vi "HFRR ADV v03.vi"() -> ()   [LabVIEW 2025] (continued)
              n1922 = local write "CH-POWER +"(w2879) -> ()
            }
            frame 12 {
              n1923 = local write "CH-POWER -"(w2880) -> ()
            }
            frame 13 {
              n1924 = local write "CH-HEATER"(w2881) -> ()
            }
            frame 14 {
              n1925 = local write "CH-HUMIDITY WET"(w2882) -> ()
            }
            frame 15 {
              n1926 = local write "CH-HUMIDITY DRY"(w2883) -> ()
            }
            frame 16 {
              n1927 = local read "Stroke PID Gains"() -> (w2886:T5)
              n1928 = Bundle By Name(cluster=w2886, "Integral Time (Ti, min)"=w2884) -> (w2885:T5)
              n1929 = local write "Stroke PID Gains"(w2885) -> ()
            }
            frame 17 {
              n1930 = local write "AIR TEMP INTERCEPT:"(w2887) -> ()
            }
            frame 18 {
              n1931 = local write "TEMP INTERCEPT:"(w2888) -> ()
            }
            frame 19 {
              n1932 = local write "S.NO"(w2889) -> ()
            }
            frame 20 {
              n1933 = local write "Com Port 3"(w2890) -> ()
            }
            frame 21 {
              n1934 = local write "LvdtOff"(w2891) -> ()
            }
            frame 22, Default {
            }
          }
        }
      }
    }
    n1935 = case shown="True" w2833 {
      frame False {
        # "79.77669138"
        # "2.3554"
        n1936 = local read "FRIC. FORCE :"() -> (w2896:dbl)
        n1937 = local read "FF cal val"() -> (w2893:dbl[])
        n1938 = Multiply(x=w2896, y=79.77669138) -> (x*y=w2895:dbl)
        n1939 = Multiply(x=w2893, y=w2895) -> (x*y=→"FF Calibration g":dbl[])
        "Err Count" <- 0 ("y")
      }
      frame True {
        n1940 = stacked-sequence {
          frame #0 {
            n1941 = stacked-sequence {
              frame #0 {
                "Lift" <- TRUE ("Lift")
              }
            }
          }
          frame #1 {
            w2908 = 2500 ("y")
            n1942 = local read "FF1"() -> (w2903:dbl[])
            n1943 = local read "Ch1"() -> (w2899:dbl[])
            "Waveform Chart 2" <- w2899
            n1944 = Array Size(array=w2903) -> (size(s)=w2902:i32)
            n1945 = Insert Into Array(array=w2903, index=w2902, new element=w2899) -> (w2905:dbl[])
            n1946 = call-poly <vilib>:"Mean.vi"("X"=w2899) -> ("mean"=→"Raw Mean":dbl)  [unwired: 1 out]
            n1947 = local read "RUN"() -> (w2900:bool)
            n1948 = Array Size(array=w2905) -> (size(s)=w2909:i32)
            n1949 = case shown="False" w2900 {
              frame False {
                n1950 = local write "Frequency"(0.0 ("Frequency")) -> ()
              }
              frame True {
              }
            }
            n1951 = Subtract(x=w2909, y=w2908) -> (x-y=w2907:i32)
            n1952 = Greater?(x=w2909, y=w2908) -> (0:w2910:bool)
            n1953 = case shown="True" w2910 {
              tunnel: w2907 -> [_ w2914]
              tunnel: [w2912 w2916] -> w2901
              tunnel: w2905 -> [w2912 w2915]
              frame False {
              }
              frame True {
                n1954 = Delete From Array(array=w2915, length=w2914, index=0) -> (array with subset deleted=w2916:dbl[])  [unwired: 1 out]
                "Numeric" <- w2914
              }
            }
            "FF1" <- w2901
            "PID Ref" <- TRUE ("PID Ref")
          }
          frame #2 {
          }
          frame #3 {
            w2917 = 0.0 ("lower limit")
            w2949 = 0.0 ("lower limit")
            # "CONVERT TO N"
            # "DATA PROCESSING"
            # "115 mV/N"
            n1955 = local read "Fric Val"() -> (w3010:dbl[])
            n1956 = local read "FRIC. FORCE :"() -> (w3000:dbl)
            n1957 = local read "Air temp"() -> (w3001:dbl[])
            n1958 = local read "temp buf"() -> (w3004:dbl[])
            n1959 = call-poly <vilib>:"Mean.vi"("X"=w3001) -> ("mean"=w2941:dbl)  [unwired: 1 out]
            "Raw air temp" <- w2941
            n1960 = local read "humid"() -> (w2951:string)
            n1961 = Multiply(x=w3010, y=1.0) -> (x*y=w3011:dbl[])
            n1962 = Multiply(x=w3000, y=79.77669138) -> (x*y=w2998:dbl)
            n1963 = call-poly <vilib>:"Mean.vi"("X"=w3004) -> ("mean"=w2943:dbl)  [unwired: 1 out]
            "Raw specimen temp" <- w2943
            n1964 = case shown="0, Default" "Calibrating" {
              tunnel: w2943 -> [w3033 _]
              tunnel: [w3033 w3034] -> w2942
              tunnel: w2941 -> [_ w3034]
              frame 0, Default {
              }
              frame 1 {
              }
            }
            n1965 = local read "HUMIDITY:"() -> (w3014:dbl)
            n1966 = Multiply(x=w3011, y=w2998) -> (x*y=w3008:dbl[])
            n1967 = Add(x=w2941, y="Offset Air Temp") -> (x+y=w2936:dbl)
            n1968 = local read "AIR TEMPERATURE :"() -> (w2985:dbl)
            n1969 = Fract/Exp String To Number(string=w2951) -> (number=w2950:dbl)  [unwired: 3 in, 1 out]
            n1970 = local read "TEMPERATURE :"() -> (w2984:dbl)
            n1971 = call-poly <vilib>:"Mean.vi"("X"=w3008) -> ("mean"=w3009:dbl)  [unwired: 1 out]
            n1972 = Multiply(x=w2950, y=w3014) -> (x*y=w3006:dbl)
            n1973 = Subtract(x=w3008, y=w3009) -> (x-y=w2947:dbl[])
            n1974 = case shown="True" "Boolean 4" {
              tunnel: w2942 -> [_ w3040]
              tunnel: "Standard Temp. ( °c )" -> [_ w3039]
              frame False {
              }
              frame True {
                n1975 = local read "Captured Values"() -> (w3037:dbl[][])
                n1976 = local write "Boolean 4"(FALSE ("Boolean 4")) -> ()
                n1977 = Build Array(w3039, w3040) -> (w3038:dbl[])
                n1978 = Build Array (concatenate)(w3037, w3038) -> (w3035:dbl[][])
                n1979 = local write "Captured Values"(w3035) -> ()
              }
            }
            n1980 = local read "AIR TEMP INTERCEPT:"() -> (w2981:dbl)
            n1981 = Multiply(x=w2936, y=w2985) -> (x*y=w2938:dbl)
            n1982 = Absolute Value(x=w2947) -> (abs(x)=w3015:dbl[])
            n1983 = Multiply(x=w2943, y=w2984) -> (x*y=w2937:dbl)
            n1984 = In Range and Coerce(upper limit=100.0, x=w3006, lower limit=w2949) -> (coerced(x)=w2953:dbl)  [unwired: 1 out]
            n1985 = local read "TEMP INTERCEPT:"() -> (w2948:dbl)
            n1986 = local read "Humid Last buf"() -> (w2976:dbl[])
            n1987 = call-poly <vilib>:"RMS.vi"("X"=w2947) -> ("rms value"=w2946:dbl)  [unwired: 1 out]
            n1988 = call-poly <vilib>:"Mean.vi"("X"=w3015) -> ()  [unwired: 2 out]
            n1989 = local read "RUN"() -> (w2997:bool)
            n1990 = Add(x=w2938, y=w2981) -> (x+y=w2983:dbl)
            n1991 = Add(x=w2937, y=w2948) -> (x+y=w2982:dbl)
            n1992 = local read "FRICVALZ"() -> (w3021:dbl)
            n1993 = Replace Array Subset(array=w2976, new element=w2953, index=0) -> (w2972:dbl[])
            n1994 = call <vilib>:"Mean PtByPt.vi"("x"=w2982, "sample length"=10) -> ("mean"=w3002:dbl)  [unwired: 2 in, 1 out]
            "TEMP 2" <- w3002
            n1995 = Select(t=0.01 ("FF fil1"), s=w2997, f=0.1 ("FF fil1")) -> (s? t:f=w2993:dbl)
            n1996 = case shown="True" "FRICVALZ 2" {
              tunnel: w2946 -> [_ w3057]
              frame False {
              }
              frame True {
                n1997 = local write "FRICVALZ 2"(FALSE ("FRICVALZ")) -> ()
                "FRICVALZ" <- w3057
              }
            }
            n1998 = Subtract(x=w2946, y=w3021) -> (x-y=w3012:dbl)
            n1999 = local read "AIR TEMP"() -> (w2990:dbl)
            n2000 = Multiply(x=w2983, y=w2993) -> (x*y=w2994:dbl)
            n2001 = Subtract(x=w2953, y=w2949) -> (x-y=w2952:dbl)
            "Humidity ( Rh )" <- w2952
            n2002 = Rotate 1D Array(1:w2972, 2:1 ("n")) -> (0:w2973:dbl[])
            n2003 = Index Array(array=w2972, index #1=0 ("index"), index #2=3 ("index")) -> (element #1=w2961:dbl, element #2=w2960:dbl)
            n2004 = case shown="True" "Boolean 5" {
              frame False {
              }
              frame True {
                n2005 = local write "Captured Values"(dbl[][] [] ("Captured Values")) -> ()
                n2006 = local write "Boolean 5"(FALSE) -> ()
                n2007 = local write "Best Fit"(dbl[] [] ("Best Fit")) -> ()
              }
            }
            n2008 = local read "FF 2"() -> (w3023:dbl)
            n2009 = Subtract(x=1.0 ("y"), y=w2993) -> (x-y=w2991:dbl)
            n2010 = Divide(x=w2961, y=w2960) -> (x/y=w2968:dbl)
            n2011 = Multiply(x=w2991, y=w2990) -> (x*y=w2989:dbl)
            n2012 = Multiply(x=w3012, y=0.1 ("FF fil1")) -> (x*y=w3027:dbl)
            n2013 = local write "TEMP"(w3002) -> ()
            n2014 = Multiply(x=0.9 ("FF fil2"), y=w3023) -> (x*y=w3026:dbl)
            n2015 = local write "Humid Last buf"(w2973) -> ()
            n2016 = Add(x=w2994, y=w2989) -> (x+y=w2987:dbl)
            n2017 = local read "offfset corr"() -> (w2964:bool)
            n2018 = local read "ecr buf"() -> (w2934:dbl[])
            n2019 = Subtract(x=1.0, y=w2968) -> (x-y=w2967:dbl)
            n2020 = Add(x=w3027, y=w3026) -> (x+y=w3020:dbl)
            "FF 2" <- w3020
            n2021 = local read "NORMAL LOAD"() -> (w3007:dbl)
            n2022 = Not A Number/Path/Refnum?(number/path/refnum=w2987) -> (NaN/Path/Refnum?=w2988:bool)
            n2023 = Absolute Value(x=w2967) -> (abs(x)=w2966:dbl)
            n2024 = Not(x=w2964) -> (.not. x?=w2962:bool)
            n2025 = Select(t=0.0, s=w2988, f=w2987) -> (s? t:f=w2919:dbl)
            "AIR TEMP" <- w2919
            n2026 = Greater Or Equal?(x=w2966, y=0.05) -> (x >= y?=w2955:bool)
            n2027 = call-poly <vilib>:"Mean.vi"("X"=w2934) -> ("mean"=w2931:dbl)  [unwired: 1 out]
            n2028 = And(x=w2955, y=w2962) -> (x .and. y?=w2963:bool)
            n2029 = Not A Number/Path/Refnum?(number/path/refnum=w2952) -> (NaN/Path/Refnum?=w3013:bool)
            n2030 = case shown="True" w3013 {
              frame False {
              }
              frame True {
                n2031 = local write "Humidity ( Rh )"(0.0 ("Humidity 3")) -> ()
              }
            }
            n2032 = case shown="True" w2963 {
              tunnel: w2961 -> [_ w3051]
              tunnel: w2960 -> [_ w3050]
              frame False {
                w3045 = 5.0 ("y")
                n2033 = local read "cnter"() -> (w3047:dbl)
                n2034 = Increment(x=w3047) -> (x+1=w3044:dbl)
                n2035 = Greater Or Equal?(x=w3044, y=w3045) -> (x >= y?=w3046:bool)
                n2036 = Select(t=w3045, s=w3046, f=w3044) -> (s? t:f=w3043:dbl)
                n2037 = local write "cnter"(w3043) -> ()
              }
              frame True {
                n2038 = Subtract(x=w3051, y=w3050) -> (x-y=→"offset":dbl)
                "offfset corr" <- TRUE ("offfset corr")
                "cnter" <- 0.0 ("cnter")
              }
            }
            n2039 = Multiply(x=w2931, y="ECR_Gain") -> (x*y=w2930:dbl)
            n2040 = local read "TEMP"() -> (w3019:dbl)
            n2041 = local read "ecr"() -> (w2925:dbl)
            n2042 = Divide(x=w3020, y=w3007) -> (x/y=w2977:dbl)
            n2043 = local read "offfset corr"() -> (w2957:bool)
            n2044 = Multiply(x=w2930, y=0.2) -> (x*y=w2923:dbl)
            n2045 = Multiply(x=0.8, y=w2925) -> (x*y=w2924:dbl)
            n2046 = call "Elapsed Time11"("Time Target (s)"=1.0) -> ("Time has Elapsed"=w2921:bool)  [unwired: 11 in, 7 out]
            n2047 = local read "cnter"() -> (w2959:dbl)
            n2048 = Not A Number/Path/Refnum?(number/path/refnum=w3019) -> (NaN/Path/Refnum?=w3018:bool)
            n2049 = Not A Number/Path/Refnum?(number/path/refnum=w3020) -> (NaN/Path/Refnum?=w3017:bool)
            n2050 = Not A Number/Path/Refnum?(number/path/refnum=w2977) -> (NaN/Path/Refnum?=w2979:bool)
            n2051 = Add(x=w2923, y=w2924) -> (x+y=w2922:dbl)
            n2052 = Select(t=0.0, s=w2979, f=w2977) -> (s? t:f=→"COF 2":dbl)
            n2053 = case shown="True" w2921 {
              tunnel: w2919 -> [_ w3029]
              frame False {
              }
              frame True {
                "AirT" <- w3029
              }
            }
            n2054 = Equal?(x=5.0 ("y"), y=w2959) -> (x = y?=w2958:bool)
            n2055 = Compound Arithmetic op=OR(w3018, w3017) -> (w3016:bool)
            n2056 = Not A Number/Path/Refnum?(number/path/refnum=w2922) -> (NaN/Path/Refnum?=w2932:bool)
            n2057 = Compound Arithmetic op=AND(w2955, w2958, w2957) -> (w2954:bool)
            n2058 = case shown="True" w3016 {
              frame False {
              }
              frame True {
                n2059 = local write "TEMP"(0.0 ("TEMP")) -> ()
                n2060 = local write "reinit"(TRUE ("reinit")) -> ()
                n2061 = local write "FF 2"(0.0 ("FF 2")) -> ()
              }
            }
            n2062 = Select(t=0.0, s=w2932, f=w2922) -> (s? t:f=w2929:dbl)
            n2063 = case shown="True" w2954 {
              frame False {
              }
              frame True {
                n2064 = local write "offfset corr"(FALSE ("offfset corr")) -> ()
                n2065 = local write "offset"(0.0 ("offset")) -> ()
              }
            }
            n2066 = In Range and Coerce(upper limit=100.0, x=w2929, lower limit=w2917) -> ()  [unwired: 2 out]
            "ecr" <- w2917
          }
          frame #4 {
            n2067 = case shown="True" "Boolean 6" {
              frame False {
              }
              frame True {
                n2068 = local read "Captured Values"() -> (w3069:dbl[][])
                n2069 = Index Array(array=w3069, index (col) #1=0 ("disabled index (col)"), index (col) #2=1 ("index (col)")) -> (element #1=w3067:dbl[], element #2=w3065:dbl[])  [unwired: 2 in]
                n2070 = local write "Boolean 6"(FALSE ("Boolean 6")) -> ()
                n2071 = call <vilib>:"Linear Fit.vi"("Y"=w3067, "X"=w3065) -> ("Best Linear Fit"=→"Best Fit":dbl[], "slope"=w3061:dbl, "intercept"=w3060:dbl)  [unwired: 9 in, 2 out]
                "Slope" <- w3061
                "Intercept" <- w3060
                n2072 = local read "Calibrating"() -> (w3062:u16)
                n2073 = case shown="1" w3062 {
                  tunnel: w3061 -> [w3071 w3073]
                  tunnel: w3060 -> [w3070 w3072]
                  frame 0, Default {
                    n2074 = local write "TEMPERATURE :"(w3071) -> ()
                    n2075 = local write "TEMP INTERCEPT:"(w3070) -> ()
                  }
                  frame 1 {
                    n2076 = local write "AIR TEMPERATURE :"(w3073) -> ()
                    n2077 = local write "AIR TEMP INTERCEPT:"(w3072) -> ()
                  }
                }
              }
            }
            n2078 = flat-sequence {
              frame #0 {
                n2079 = Wait (ms)(milliseconds to wait=u32 100) -> ()  [unwired: 1 out]
              }
              frame #1 {
                n2080 = local write "Lift"(FALSE ("Lift")) -> ()
              }
            }
          }
        }
      }
    }
    n2081 = local read "EXIT"() -> (w2840:bool)
    "Rate" <- 2500.0 ("No of Samples")
    "Humid Last buf" <- dbl[] [0.0, 0.0, 0.0, 0.0] ("Humid Last buf")
  }
  n2082 = VISA Close(VISA resource name=w19, error in (no error)=w18) -> (error out=w20:errorcluster)
  n2083 = call <vilib>:"Clear Errors.vi"("error in (no error)"=w20) -> ()  [unwired: 5 in, 2 out]
  n2084 = VISA Close(VISA resource name=w47, error in (no error)=w46) -> (error out=w44:errorcluster)
  n2085 = call <vilib>:"Clear Errors.vi"("error in (no error)"=w44) -> ()  [unwired: 5 in, 2 out]
  n2086 = Or(x=w34, y=w33) -> (x .or. y?=w35:bool)
  n2087 = while {
    tunnel: [w3135] -> w40
    shift-right: [w3115] -> _
    shift-left: "" -> [w3103]
    tunnel: [w3091] -> _
    i -> [w3091]
    stop <- w3135 stop-if-true
    w3117 = ";" ("string")
    n2088 = local read "start en"() -> (w3137:bool)
    n2089 = And(x="st enable", y=w3137) -> (x .and. y?=w3138:bool)
    n2090 = local read "ACQUIRE 3"() -> (w3080:bool)
    n2091 = local read "Elapsed time"() -> (w3099:dbl)
    n2092 = case shown="True" w3138 {
      tunnel: "st enable" -> [w3202 w3203]
      tunnel: [w3202 w3203] -> w3081
      frame False {
      }
      frame True {
        n2093 = local write "start en"(FALSE ("start en")) -> ()
      }
    }
    n2094 = Wait (ms)(milliseconds to wait=u32 80) -> ()  [unwired: 1 out]
    n2095 = local read "Stroke"() -> (w3090:dbl)
    n2096 = Greater?(x=w3099, y=0.1) -> (0:w3097:bool)
    n2097 = Or(x=w3081, y=w3080) -> (x .or. y?=w3082:bool)
    n2098 = case shown="True" "ACQUIRE 2" {
      frame False {
      }
      frame True {
        n2099 = call "Elapsed Time13"() -> ("Time has Elapsed"=w3145:bool)  [unwired: 12 in, 7 out]
        n2100 = case shown="True" w3145 {
          frame False {
          }
          frame True {
            n2101 = local write "ACQUIRE 2"(FALSE ("ACQUIRE 2")) -> ()
            n2102 = local write "ACQUIRE 3"(FALSE ("ACQUIRE 2")) -> ()
          }
        }
        n2103 = local write "ACQUIRE 3"(TRUE ("ACQUIRE 2")) -> ()
      }
    }
    n2104 = case shown="True" w3082 {
      tunnel: w3090 -> [_ w3225]
      tunnel: [w3205 _] -> w3134
      tunnel: w3097 -> [_ _]
      tunnel: w3080 -> [_ w3212]
      frame False {
        w3205 = TRUE ("PID Rst")
        n2105 = local read "stop cmd"() -> (w3206:bool)
        n2106 = case shown="True" w3206 {
          frame False {
          }
          frame True {
            n2107 = local write "stop cmd"(FALSE ("stop cmd")) -> ()
          }
        }
        n2108 = local write "PID Rst"(TRUE ("PID Rst")) -> ()
        "start en" <- w3205
      }
      frame True {
        w3232 = cluster{"output high":dbl, "output low":dbl} {"output high"=600.0, "output low"=-600.0} ("output range")
        n2109 = local read "STROKE GAIN :"() -> (w3217:dbl)
        n2110 = call "Elapsed Time6"("Reset"="PID Rst", "Auto Reset"=FALSE) -> ("Time has Elapsed"=w3226:bool)  [unwired: 10 in, 7 out]
        n2111 = Multiply(x="Set Strk", y=w3217) -> (x*y=w3210:dbl)
        n2112 = case shown="False" w3226 {
          tunnel: [w3237 w3238] -> w3229
          tunnel: "Set Strk" -> [w3237 _]
          tunnel: w3225 -> [_ w3238]
          frame False {
          }
          frame True {
          }
        }
        n2113 = Multiply(x=w3210, y=1.0) -> (x*y=w3209:dbl)
        n2114 = Select(t=T5 {"Proportional Gain (Kc)"=0.0, "Integral Time (Ti, min)"=0.02, "Derivative Time (Td, min)"=0.0} ("Stroke PID Gains"), s=w3212, f="Stroke PID Gains") -> (s? t:f=w3213:T5)
        n2115 = Not(x=w3226) -> (.not. x?=w3224:bool)
        n2116 = call-poly <vilib>:"PID.vi"("reinitialize? (F)"=w3224, "output range"=w3232, "PID gains"=w3213, "process variable"=w3229, "setpoint"="Set Strk") -> ("output"=w3223:dbl)  [unwired: 5 in, 1 out]
        "Slide 5" <- w3223
        n2117 = Select(t=w3223, s=w3226, f=0.0) -> (s? t:f=w3227:dbl)
        n2118 = flat-sequence {
          tunnel: w3227 -> [_]
          frame #0 {
            n2119 = local write "PID Rst"(FALSE ("PID Rst")) -> ()
          }
        }
        n2120 = Add(x=w3209, y=w3227) -> (x+y=w3222:dbl)
        n2121 = Unbundle(w3232) -> ("output high"=w3231:dbl, "output low"=w3230:dbl)
        n2122 = To Word Integer(number=w3222) -> (16bit integer=w3219:i16)
        n2123 = property on="Slide 5" class="Slide (strict)"("Scale.Range:Minimum"=w3230, "Scale.Range:Maximum"=w3231) -> ()  [unwired: 2 in, 2 out]
        n2124 = In Range and Coerce(upper limit=4095.0 ("f"), x=w3219, lower limit=100.0 ("f")) -> (coerced(x)=w3216:dbl)  [unwired: 1 out]
        "PID Out" <- w3216
        n2125 = Number To Decimal String(number=w3216) -> (decimal integer string=→"st gain":string)  [unwired: 1 in]
        "stop cmd" <- TRUE ("Auto Reset")
      }
    }
    n2126 = flat-sequence {
      frame #0 {
        n2127 = local read "CH-POWER +"() -> (w3149:u16)
        n2128 = local read "CH-POWER -"() -> (w3150:u16)
        n2129 = case shown="1" w3150 {
          tunnel: "PWR" -> [w3151 w3152 w3153 w3154 w3155 w3156 w3157 w3158]
          frame 0, Default {
            n2130 = local write "Do 0"(w3151) -> ()
          }
          frame 1 {
            n2131 = local write "Do 1"(w3152) -> ()
          }
          frame 2 {
            n2132 = local write "Do 2"(w3153) -> ()
          }
          frame 3 {
            n2133 = local write "Do 3"(w3154) -> ()
          }
          frame 4 {
            n2134 = local write "Do 4"(w3155) -> ()
          }
          frame 5 {
            n2135 = local write "Do 5"(w3156) -> ()
          }
          frame 6 {
            n2136 = local write "Do 6"(w3157) -> ()
          }
          frame 7 {
            n2137 = local write "Do 7"(w3158) -> ()
          }
        }
        n2138 = case shown="1" w3149 {
          tunnel: "PWR" -> [w3159 w3160 w3161 w3162 w3163 w3164 w3165 w3166]
          frame 0, Default {
            n2139 = local write "Do 0"(w3159) -> ()
          }
          frame 1 {
            n2140 = local write "Do 1"(w3160) -> ()
          }
          frame 2 {
            n2141 = local write "Do 2"(w3161) -> ()
          }
          frame 3 {
            n2142 = local write "Do 3"(w3162) -> ()
          }
          frame 4 {
            n2143 = local write "Do 4"(w3163) -> ()
          }
          frame 5 {
            n2144 = local write "Do 5"(w3164) -> ()
          }
          frame 6 {
            n2145 = local write "Do 6"(w3165) -> ()
          }
          frame 7 {
            n2146 = local write "Do 7"(w3166) -> ()
          }
        }
      }
    }
    n2147 = local read "RUN"() -> (w3088:bool)
    n2148 = Or(x=w3088, y="ACQUIRE 3") -> (x .or. y?=w3087:bool)
    n2149 = local read "Set Hz"() -> (w3105:dbl)
    n2150 = Select(t=w3105, s=w3087, f=0.0) -> (s? t:f=w3104:dbl)
    n2151 = local read "st gain"() -> (w3108:string)
    n2152 = local read "DO"() -> (w3109:string)
    n2153 = case shown="True" "Boolean 10" {
      frame False {
      }
      frame True {
        n2154 = local write "Tab Control 8"(enum32{"setup", "calibrate"}."calibrate" ("Tab Control 8")) -> ()
        n2155 = local write "Boolean 10"(FALSE ("Boolean 10")) -> ()
      }
    }
    n2156 = Number To Decimal String(number=w3104) -> (decimal integer string=w3107:string)  [unwired: 1 in]
    n2157 = case shown="True" "Boolean 11" {
      frame False {
      }
      frame True {
        n2158 = local write "Tab Control 8"(enum32{"setup", "calibrate"}."setup" ("Tab Control 8")) -> ()
        n2159 = local write "Boolean 11"(FALSE ("Boolean 11")) -> ()
      }
    }
    n2160 = String Length(string=w3108) -> (length=w3123:i32)
    n2161 = String Length(string=w3109) -> (length=w3111:i32)
    n2162 = String Length(string=w3107) -> (length=w3124:i32)
    n2163 = Subtract(x=4.0, y=w3123) -> (x-y=w3120:dbl)
    n2164 = Subtract(x=3.0, y=w3111) -> (x-y=w3114:dbl)
    n2165 = flat-sequence {
      tunnel: w3134 -> [_]
      frame #0 {
        n2166 = Build Array("Do 0", "Do 1", "Do 2", "Do 3", "Do 4", "Do 5", "Do 6", "Do 7") -> (w3193:bool[])
        n2167 = Boolean Array To Number(Boolean array=w3193) -> (number=w3191:u32)
        n2168 = Add(x=w3191, y=u32 0) -> (x+y=w3189:u32)
        n2169 = Number To Decimal String(number=w3189) -> (decimal integer string=→"DO":string)  [unwired: 1 in]
      }
    }
    n2170 = Subtract(x=3.0, y=w3124) -> (x-y=w3125:dbl)
    n2171 = Replace Substring(3:w3120, 4:w3108, 5:"0000" ("string")) -> (1:w3118:string)  [unwired: 1 in, 1 out]
    n2172 = Replace Substring(3:w3114, 4:w3109, 5:"000" ("string")) -> (1:w3110:string)  [unwired: 1 in, 1 out]
    n2173 = Replace Substring(3:w3125, 4:w3107, 5:"000" ("string")) -> (1:w3119:string)  [unwired: 1 in, 1 out]
    n2174 = Concatenate Strings("*" ("string"), w3119, w3117, w3118, w3117, w3110, "$" ("string")) -> (w3115:string)
    "Stroke_send_Val" <- w3115
    n2175 = local read "RUN"() -> (w3085:bool)
    n2176 = local read "ACQUIRE 3"() -> (w3084:bool)
    n2177 = local read "send"() -> (w3101:bool)
    n2178 = Not Equal?(x=w3103, y=w3115) -> (x != y?=w3116:bool)
    n2179 = Or(x=w3085, y=w3084) -> (x .or. y?=w3083:bool)
    n2180 = And(x=w3101, y=w3083) -> (x .and. y?=w3100:bool)
    n2181 = Or(x=w3116, y=w3100) -> (x .or. y?=w3094:bool)
    n2182 = case shown="False" w3083 {
      frame False {
        "send" <- TRUE ("send")
      }
      frame True {
      }
    }
    n2183 = call "Elapsed Time4"("Time Target (s)"=0.5) -> ("Time has Elapsed"=w3092:bool)  [unwired: 11 in, 7 out]
    n2184 = local read "Din"() -> (w3133:u8[])
    n2185 = Or(x=w3092, y=w3094) -> (x .or. y?=w3093:bool)
    n2186 = Index Array(array=w3133, index=0) -> (element=w3131:u8)
    n2187 = case shown="True" w3093 {
      tunnel: w3115 -> [_ w3170]
      frame False {
      }
      frame True {
        n2188 = local read "Due Com"() -> (w3171:string[])
        n2189 = Build Array (concatenate)(w3171, w3170) -> (→"Due Com":string[])
        n2190 = local write "send"(FALSE ("send")) -> ()
      }
    }
    n2191 = Number To Boolean Array(number=w3131) -> (Boolean array=w3130:bool[])
    n2192 = Array Size(array=w3130) -> (size(s)=w3129:i32)
    n2193 = Greater Than 0?(x=w3129) -> (x > 0?=w3128:bool)
    n2194 = case shown="True" w3128 {
      tunnel: w3130 -> [_ w3185]
      frame False {
      }
      frame True {
        n2195 = Index Array(array=w3185, index #1=0 ("index"), index #2=1 ("index"), index #3=2 ("index"), index #4=3 ("index"), index #5=4 ("index"), index #6=5 ("index"), index #7=6 ("index"), index #8=7 ("index")) -> (element #1=→"DI 0":bool, element #2=→"DI 1":bool, element #3=→"DI 2":bool, element #4=→"DI 3":bool, element #5=→"DI 4":bool, element #6=→"DI 5":bool, element #7=→"DI 6":bool, element #8=→"DI 7":bool)
      }
    }
    n2196 = local read "EXIT"() -> (w3135:bool)
  }
  n2197 = Or(x=w25, y=w35) -> (x .or. y?=w42:bool)
  n2198 = control-ref of="new picture"() -> ()  [unwired: 1 out]
  n2199 = Or(x=w49, y=w42) -> (x .or. y?=w39:bool)
  n2200 = Or(x=w39, y=w40) -> (x .or. y?=w28:bool)
  n2201 = while {
    tunnel: w23 -> [_]
    tunnel: [w3241] -> w53
    tunnel: [w3240] -> _
    i -> [w3240]
    stop <- w3241 stop-if-true
    n2202 = local read "PID-out"() -> (w3242:dbl)
    "Horizontal Slider Control" <- w3242
    n2203 = Greater Or Equal?(x=w3242, y=2.0) -> (x >= y?=w3243:bool)
    n2204 = flat-sequence {
      tunnel: w3243 -> [w3251]
      tunnel: w3242 -> [w3254]
      tunnel: [w3252] -> w3249
      tunnel: [w3250] -> w3248
      tunnel: [w3270] -> w3247
      tunnel: w3249 -> [w3270]
      tunnel: w3248 -> [w3267]
      tunnel: [w3267] -> w3246
      tunnel: w3247 -> [w3272]
      tunnel: [w3271] -> w3245
      tunnel: w3246 -> [w3271]
      tunnel: w3245 -> [w3286]
      frame #0 {
        n2205 = case shown="True" w3251 {
          selector: w3251 -> [w3256 _]
          frame False {
            n2206 = local write "HEATER"(w3256) -> ()
          }
          frame True {
            w3258 = TRUE ("data")
            n2207 = local read "CH-HEATER"() -> (w3257:u16)
            n2208 = case shown="2" w3257 {
              tunnel: w3258 -> [w3259 w3260 w3261 w3262 w3263 w3264 w3265 w3266]
              frame 0, Default {
                n2209 = local write "Do 0"(w3259) -> ()
              }
              frame 1 {
                n2210 = local write "Do 1"(w3260) -> ()
              }
              frame 2 {
                n2211 = local write "Do 2"(w3261) -> ()
              }
              frame 3 {
                n2212 = local write "Do 3"(w3262) -> ()
              }
              frame 4 {
                n2213 = local write "Do 4"(w3263) -> ()
              }
              frame 5 {
                n2214 = local write "Do 5"(w3264) -> ()
              }
              frame 6 {
                n2215 = local write "Do 6"(w3265) -> ()
              }
              frame 7 {
                n2216 = local write "Do 7"(w3266) -> ()
              }
            }
            "HEATER" <- w3258
          }
        }
        n2217 = Select(t=w3254, s=w3251, f=0.0) -> (s? t:f=w3250:dbl)
        n2218 = Greater Or Equal?(x=w3254, y=97.0) -> (x >= y?=w3252:bool)
      }
      frame #1 {
        n2219 = Multiply(x=w3267, y=5.0) -> (x*y=w3269:dbl)
        n2220 = Wait (ms)(milliseconds to wait=w3269) -> ()  [unwired: 1 out]
      }
      frame #2 {
        n2221 = case shown="True" w3272 {
          frame False {
            w3273 = FALSE ("data")
            n2222 = local write "HEATER"(w3273) -> ()
            n2223 = local read "CH-HEATER"() -> (w3274:u16)
            n2224 = case shown="4" w3274 {
              tunnel: w3273 -> [w3275 w3276 w3277 w3278 w3279 w3280 w3281 w3282]
              frame 0, Default {
                n2225 = local write "Do 0"(w3275) -> ()
              }
              frame 1 {
                n2226 = local write "Do 1"(w3276) -> ()
              }
              frame 2 {
                n2227 = local write "Do 2"(w3277) -> ()
              }
              frame 3 {
                n2228 = local write "Do 3"(w3278) -> ()
              }
              frame 4 {
                n2229 = local write "Do 4"(w3279) -> ()
              }
              frame 5 {
                n2230 = local write "Do 5"(w3280) -> ()
              }
              frame 6 {
                n2231 = local write "Do 6"(w3281) -> ()
              }
              frame 7 {
                n2232 = local write "Do 7"(w3282) -> ()
              }
            }
          }
          frame True {
          }
        }
      }
      frame #3 {
        n2233 = Subtract(x=100, y=w3286) -> (x-y=w3285:dbl)
        n2234 = Multiply(x=w3285, y=5.0) -> (x*y=w3283:dbl)
        n2235 = Wait (ms)(milliseconds to wait=w3283) -> ()  [unwired: 1 out]
      }
    }
    n2236 = local read "EXIT"() -> (w3241:bool)
  }
  n2237 = while {
    shift-right: [w3329] -> w16
    shift-left: errorcluster {"status"=TRUE, "code"=0, "source"="Init"} ("error out") -> [w3293]
    shift-right: [w3328] -> w15
    shift-left: _ -> [w3294]
    shift-right: [w3327] -> _
    shift-left: "" -> [w3326]
    tunnel: [w3325] -> w29
    shift-right: ["Set Rh"] -> _
    shift-left: 0.0 ("Set Rh") -> [w3319]
    tunnel: [w3296] -> _
    i -> [w3296]
    stop <- w3325 stop-if-true
    n2238 = local read "Com Port 3"() -> (w3295:refnum<visa-resource-name>)
    n2239 = flat-sequence {
      tunnel: w3293 -> [w3332]
      tunnel: [w3332] -> w3292
      frame #0 {
        n2240 = Wait (ms)(milliseconds to wait=u32 200) -> ()  [unwired: 1 out]
      }
    }
    n2241 = Not Equal?(x=w3295, y=w3294) -> (x != y?=w3290:bool)
    n2242 = Or(x=w3290, y="Re-Initialise") -> (x .or. y?=w3289:bool)
    n2243 = case shown="True" w3289 {
      tunnel: w3292 -> [w3330 _]
      tunnel: [w3330 errorcluster {"status"=TRUE, "code"=0, "source"="Init"} ("error out")] -> w3291
      frame False {
      }
      frame True {
      }
    }
    n2244 = case shown="Error" w3291 {
      selector: w3291 -> [w3357 w3403]
      tunnel: [w3355 w3396] -> w3329
      tunnel: w3294 -> [w3358 w3402]
      tunnel: [w3356 w3405] -> w3328
      tunnel: w3326 -> [w3345 w3404]
      tunnel: [w3352 w3404] -> w3327
      frame No Error {
        n2245 = call "Elapsed Time7"() -> ("Time has Elapsed"=w3351:bool)  [unwired: 12 in, 7 out]
        n2246 = Not Equal?(x="Humidity Str Send", y=w3345) -> (x != y?=w3347:bool)
        n2247 = Or(x=w3347, y=w3351) -> (x .or. y?=w3350:bool)
        n2248 = Select(t="Humidity Str Send", s=w3347, f="vals" ("regular expression")) -> (s? t:f=w3346:string)
        n2249 = Or(x=w3350, y="Send") -> (x .or. y?=w3354:bool)
        n2250 = case shown="True" w3354 {
          tunnel: [w3361 w3366] -> w3355
          tunnel: w3358 -> [w3360 w3374]
          tunnel: w3357 -> [w3361 w3373]
          tunnel: [w3360 w3367] -> w3356
          tunnel: w3346 -> [_ w3372]
          tunnel: [w3359 w3363] -> w3352
          tunnel: "Humidity Str Send" -> [_ w3364]
          tunnel: w3347 -> [_ w3365]
          tunnel: w3345 -> [w3359 w3362]
          frame False {
          }
          frame True {
            n2251 = flat-sequence {
              tunnel: w3374 -> [w3382]
              tunnel: w3373 -> [w3381]
              tunnel: w3372 -> [w3378]
              tunnel: [w3380] -> w3371
              tunnel: [w3379] -> w3370
              tunnel: w3371 -> [w3385]
              tunnel: w3370 -> [w3384]
              tunnel: [w3385] -> w3369
              tunnel: [w3384] -> w3368
              tunnel: w3369 -> [w3392]
              tunnel: w3368 -> [w3391]
              tunnel: [w3390] -> w3367
              tunnel: [w3389] -> w3366
              frame #0 {
                n2252 = Concatenate Strings(w3378, "\r") -> (w3377:string)
                n2253 = local write "Ser Led"(TRUE ("Boolean 4")) -> ()
                n2254 = VISA Write(VISA resource name=w3382, write buffer=w3377, error in (no error)=w3381) -> (VISA resource name out=w3380:refnum<visa-resource-name>, error out=w3379:errorcluster)  [unwired: 1 out]
              }
              frame #1 {
                n2255 = Wait (ms)(milliseconds to wait="wait") -> ()  [unwired: 1 out]
              }
              frame #2 {
                w3387 = FALSE ("Send")
                n2256 = property class="Instr"(reference=w3392, error in=w3391) -> (reference out=w3393:refnum<visa-resource-name>, error out=w3394:errorcluster, "Serial Settings:Number of Bytes at Serial Port"=w3386:u32)
                "Humidity 2" <- w3386
                n2257 = VISA Read(VISA resource name=w3393, byte count=w3386, error in (no error)=w3394) -> (VISA resource name out=w3390:refnum<visa-resource-name>, read buffer=→"Humidity Str Rec":string, error out=w3389:errorcluster)  [unwired: 1 out]
                n2258 = local write "Ser Led"(w3387) -> ()
                n2259 = local write "Send"(w3387) -> ()
              }
            }
            n2260 = Select(t=w3364, s=w3365, f=w3362) -> (s? t:f=w3363:string)
          }
        }
      }
      frame Error {
        w3410 = u16 0 items=["None"=0, "XON/XOFF"=1, "RTS/CTS"=2, "DTR/DSR"=4] ("flow control")
        w3406 = u16 0 items=["None", "Odd", "Even", "Mark", "Space"] ("parity")
        w3409 = u16 10 items=["1.0"=10, "1.5"=15, "2.0"=20] ("stop bits")
        n2261 = VISA Close(VISA resource name=w3402, error in (no error)=w3403) -> (error out=w3401:errorcluster)
        n2262 = local write "Humidity Str Rec"("" ("Humidity Str Rec")) -> ()
        n2263 = call <vilib>:"Clear Errors.vi"("error in (no error)"=w3401) -> ("error out"=w3400:errorcluster)  [unwired: 5 in, 1 out]
        n2264 = local read "Com Port 3"() -> (w3399:refnum<visa-resource-name>)
        n2265 = local write "humid"("" ("humid")) -> ()
        n2266 = call-poly "VISA Configure Serial Port"("VISA resource name"=w3399, "timeout (10sec)"=u32 1000, "termination char\n(0xA = '\\n' = LF)"=u8 10 ("termination char\n(0xA = '\\n' = LF)"), "Enable Termination\nChar (T)"=FALSE ("Enable Termination Char (T)"), "baud rate (9600)"="Humidity BaudRate", "data bits (8)"=u16 8 ("data bits"), "parity (0:none)"=w3406, "error in (no error)"=w3400, "stop bits (10: 1 bit)"=w3409, "flow control (0:none)"=w3410) -> ("VISA resource name out"=w3405:refnum<visa-resource-name>, "error out"=w3396:errorcluster)  [unwired: 4 in]
        "Port 3 Error" <- w3396
      }
    }
    n2267 = local read "Humidity Str Rec"() -> (w3297:string)
    n2268 = String Subset(string=w3297, offset (0)=7) -> (substring=w3312:string)  [unwired: 1 in]
    n2269 = Match Pattern(string=w3312, regular expression="g") -> (after substring=w3313:string, offset past match=w3304:i32)  [unwired: 1 in, 2 out]
    n2270 = Match Pattern(string=w3312, regular expression="y") -> (after substring=w3311:string, offset past match=w3305:i32)  [unwired: 1 in, 2 out]
    n2271 = Match Pattern(string=w3297, regular expression="v") -> (offset past match=w3318:i32)  [unwired: 1 in, 3 out]
    n2272 = Match Pattern(string=w3297, regular expression="?") -> (offset past match=w3315:i32)  [unwired: 1 in, 3 out]
    n2273 = Number To Decimal String(number="Set Rh") -> (decimal integer string=w3322:string)  [unwired: 1 in]
    n2274 = Greater Or Equal To 0?(x=w3305) -> (x >= 0?=w3302:bool)
    n2275 = Greater Or Equal To 0?(x=w3304) -> (x >= 0?=w3303:bool)
    n2276 = Greater Or Equal To 0?(x=w3318) -> (x >= 0?=w3300:bool)
    n2277 = Equal?(x=w3315, y=-1) -> (x = y?=w3299:bool)
    n2278 = Not Equal?(x="Set Rh", y=w3319) -> (x != y?=w3324:bool)
    n2279 = Greater?(x=w3305, y=w3304) -> (0:w3310:bool)
    n2280 = Or(x=w3302, y=w3303) -> (x .or. y?=w3301:bool)
    n2281 = Compound Arithmetic op=AND(w3300, w3299, w3301) -> (w3298:bool)
    n2282 = Concatenate Strings("#setPoint00" ("string"), w3322) -> (w3323:string)
    n2283 = Select(t=w3311, s=w3310, f=w3313) -> (s? t:f=w3306:string)
    n2284 = case shown="True" w3298 {
      tunnel: w3297 -> [_ _]
      tunnel: w3306 -> [_ w3337]
      frame False {
      }
      frame True {
        w3335 = " " ("regular expression")
        n2285 = Match Pattern(string=w3337, regular expression=" ") -> (after substring=w3339:string)  [unwired: 1 in, 3 out]
        n2286 = Match Pattern(string=w3339, regular expression=w3335) -> (before substring=→"humid":string, after substring=w3336:string)  [unwired: 1 in, 2 out]
        n2287 = Match Pattern(string=w3336, regular expression=w3335) -> (before substring=→"temp_@Rh sensor":string)  [unwired: 1 in, 3 out]
      }
    }
    n2288 = case shown="False" w3324 {
      tunnel: w3323 -> [_ w3344]
      frame False {
        n2289 = local read "Humidity"() -> (w3341:bool)
        n2290 = case shown="True" w3341 {
          frame False {
            n2291 = local write "Humidity Str Send"("stop" ("Humidity Str Send")) -> ()
          }
          frame True {
            n2292 = local write "Humidity Str Send"("start" ("Humidity Str Send")) -> ()
          }
        }
      }
      frame True {
        n2293 = local write "Humidity Str Send"(w3344) -> ()
      }
    }
    n2294 = local read "EXIT"() -> (w3325:bool)
  }
  n2295 = VISA Close(VISA resource name=w15, error in (no error)=w16) -> (error out=w26:errorcluster)
  n2296 = call <vilib>:"Clear Errors.vi"("error in (no error)"=w26) -> ()  [unwired: 5 in, 2 out]
  n2297 = Or(x=w28, y=w29) -> (x .or. y?=w27:bool)
  n2298 = Or(x=w53, y=w27) -> (x .or. y?=w52:bool)
  n2299 = while {
    tunnel: [w3419] -> _
    tunnel: w23 -> [_]
    i -> [w3419]
    stop <- w3418 stop-if-true
    # "Langauage selection"
    n2300 = property on="FF Calibration g" class="WFGraph (strict)"("Plot Area:Colors:FG Color"=u32 0) -> ()  [unwired: 2 in, 2 out]
    n2301 = Equal?(x="Lan flag", y=22.0) -> ()  [unwired: 1 out]
    n2302 = case shown="True" "Case Constant\n(See Context Help) 5" {
      frame False {
      }
      frame True {
        n2303 = stacked-sequence {
          frame #0 {
            n2304 = case shown="\"Russian\"" "Language Selection" {
              tunnel: [0 1] -> w3421
              frame "English", Default {
              }
              frame "Russian" {
              }
            }
            n2305 = for {
              N: 130 -> [_]
              tunnel: "Table" -> [w3430]
              tunnel: w3421 -> [w3429]
              i -> [w3428]
              n2306 = Index Array(array=w3430, index (row)=w3428, index (col)=w3429) -> (element=w3427:string)
              n2307 = case shown="8" w3428 {
                tunnel: w3427 -> [w3431 w3432 w3433 w3434 w3435 w3436 w3437 w3438 w3439 w3440 w3441 w3442 w3443 w3444 w3445 w3446 w3447 w3448 w3449 w3450 w3451 w3452 w3453 w3454 w3455 w3456 w3457 w3458 w3459 _ _ w3460 w3461 w3462 w3463 w3464 w3465 w3474 w3481 w3488 w3495 w3499 w3502 w3505 w3507 w3509 w3510 w3511 w3512 w3513 w3514 w3515 w3516 w3517 w3518 w3519 w3520 w3521 w3522 w3523 w3524 w3525 w3526 w3527 w3528 w3529 w3530 w3531 w3532 w3533 w3534 w3535 w3536 w3537 w3538 w3539 w3540 w3541 w3542 w3543 w3544 w3545 w3546 w3547 w3548 w3549 w3550 w3551 w3552 w3553 w3554 w3555 w3556 w3557 w3558 w3559 w3560 w3561 w3562 w3563 w3564 w3565 w3566 w3567 w3568 _ w3569 w3570 w3571 w3572 w3573 w3574 w3575 w3576 w3577 w3578 w3579 w3580 w3581 _ w3582 w3583 w3584 w3585 w3586 w3587 _]
                frame 0 {
                  n2308 = local write "S"(w3431) -> ()
                }
                frame 1 {
                  n2309 = local write "S 2"(w3432) -> ()
                }
                frame 2 {
                  n2310 = property on="EXIT" class="Bool (strict)"("Boolean Text.Text"=w3433) -> ()  [unwired: 2 in, 2 out]
                }
                frame 3 {
                  n2311 = local write "S 4"(w3434) -> ()
                }
                frame 4 {
                  n2312 = property on="FILE" class="Str"("Caption.Text"=w3435) -> ()  [unwired: 2 in, 2 out]
                }
                frame 5 {
                  n2313 = property on="Fuel Discription :" class="Str"("Caption.Text"=w3436) -> ()  [unwired: 2 in, 2 out]
                }
                frame 6 {
                  n2314 = property on="Remarks :" class="Str"("Caption.Text"=w3437) -> ()  [unwired: 2 in, 2 out]
                }
                frame 7 {
                  n2315 = property on="Save & Continue" class="Bool (strict)"("Boolean Text.Text"=w3438) -> ()  [unwired: 2 in, 2 out]
                }
                frame 8 {
                  n2316 = property on="STOP 3" class="Bool (strict)"("Boolean Text.Text"=w3439) -> ()  [unwired: 2 in, 2 out]
                }
                frame 9 {
                  n2317 = property on="Set Hz" class="DigNum (strict)"("Caption.Text"=w3440) -> ()  [unwired: 2 in, 2 out]
                }
                frame 10 {
                  "String 3" <- w3441
                }
                frame 11 {
                  n2318 = property on="NORMAL LOAD" class="DigNum (strict)"("Caption.Text"=w3442) -> ()  [unwired: 2 in, 2 out]
                }
                frame 12 {
                  "String 5" <- w3443
                }
                frame 13 {
                  n2319 = property on="Set Temp" class="DigNum (strict)"("Caption.Text"=w3444) -> ()  [unwired: 2 in, 2 out]
                }
                frame 14 {
                  n2320 = local write "S 15"(w3445) -> ()
                }
                frame 15 {
                  n2321 = property on="Set Rh" class="DigNum (strict)"("Caption.Text"=w3446) -> ()  [unwired: 2 in, 2 out]
                }
                frame 16 {
                  "String 13" <- w3447
                  "String 26" <- w3447
                }
                frame 17 {
                  n2322 = local write "S 18"(w3448) -> ()
                }
                frame 18 {
                  "String 17" <- w3449
                }
                frame 19 {
                  n2323 = property on="test time" class="DigNum (strict)"("Caption.Text"=w3450) -> ()  [unwired: 2 in, 2 out]
                }
                frame 20 {
                  "String 18" <- w3451
                  "String 22" <- w3451
                }
                frame 21 {
                  n2324 = property on="Elapsed time" class="DigNum (strict)"("Caption.Text"=w3452) -> ()  [unwired: 2 in, 2 out]
                }
                frame 22 {
                  n2325 = property on="Samplingtime 2" class="DigNum (strict)"("Caption.Text"=w3453) -> ()  [unwired: 2 in, 2 out]
                }
                frame 23 {
                  "String 21" <- w3454
                }
                frame 24 {
                  n2326 = property on="Countdown" class="DigNum (strict)"("Caption.Text"=w3455) -> ()  [unwired: 2 in, 2 out]
                }
                frame 25 {
                  n2327 = property on="Countdown 2" class="DigNum (strict)"("Caption.Text"=w3456) -> ()  [unwired: 2 in, 2 out]
                }
                frame 26 {
                  n2328 = property on="Engage" class="Bool (strict)"("Boolean Text.Text"=w3457) -> ()  [unwired: 2 in, 2 out]
                }
                frame 27 {
                  n2329 = property on="Boolean  4" class="Bool (strict)"("Boolean Text.Text"=w3458) -> ()  [unwired: 2 in, 2 out]
                }
                frame 28 {
                  n2330 = property on="Test \nStatus" class="Bool (strict)"("Boolean Text.Text"=w3459) -> ()  [unwired: 2 in, 2 out]
                }
                frame 29 {
                }
                frame 30 {
                }
                frame 31 {
                  n2331 = property on="FF Calibration g" class="WFGraph (strict)"("X Scale.Name Label.Text"=w3460) -> ()  [unwired: 2 in, 2 out]
                }
                frame 32 {
                  n2332 = property on="RSTCOF" class="Bool"("Boolean Text.Text"=w3461) -> ()  [unwired: 2 in, 2 out]
                  n2333 = property on="RST FF" class="Bool"("Boolean Text.Text"=w3461) -> ()  [unwired: 2 in, 2 out]
                  n2334 = property on="RST TEMP" class="Bool"("Boolean Text.Text"=w3461) -> ()  [unwired: 2 in, 2 out]
                  n2335 = property on="RSTV1 3" class="Bool"("Boolean Text.Text"=w3461) -> ()  [unwired: 2 in, 2 out]
                  n2336 = property on="rstv2" class="Bool"("Boolean Text.Text"=w3461) -> ()  [unwired: 2 in, 2 out]
                  n2337 = property on="RSTV1 2" class="Bool"("Boolean Text.Text"=w3461) -> ()  [unwired: 2 in, 2 out]
                  n2338 = property on="RST CP" class="Bool"("Boolean Text.Text"=w3461) -> ()  [unwired: 2 in, 2 out]
                }
                frame 33 {
                  "S 61" <- w3462
                }
                frame 34 {
                  "String 23" <- w3463
                }
                frame 35 {
                  n2339 = property on="Rh Before" class="DigNum (strict)"("Caption.Text"=w3464) -> ()  [unwired: 2 in, 2 out]
                }
                frame 36 {
                  n2340 = Match Pattern(string=w3465, regular expression=",") -> (before substring=→"bs":string, after substring=→"as":string)  [unwired: 1 in, 2 out]
                  n2341 = property on="Rh After" class="DigNum (strict)"("Caption.Text"=w3465) -> ()  [unwired: 2 in, 2 out]
                }
                frame 37 {
                  n2342 = Match Pattern(string=w3474, regular expression=",") -> (before substring=w3473:string, after substring=w3472:string)  [unwired: 1 in, 2 out]
                  "bs" <- w3473
                  "as" <- w3472
                  n2343 = Concatenate Strings(w3473, w3472) -> (w3469:string)
                  n2344 = property on="Humidity before test 2" class="DigNum (strict)"("Caption.Text"=w3469) -> ()  [unwired: 2 in, 2 out]
                  n2345 = property on="Humidity before test" class="DigNum (strict)"("Caption.Text"=w3469) -> ()  [unwired: 2 in, 2 out]
                  n2346 = Concatenate Strings(w3469, "=" ("string")) -> (w3470:string)
                  n2347 = local write "S 38"(w3470) -> ()
                }
                frame 38 {
                  n2348 = Match Pattern(string=w3481, regular expression=",") -> (before substring=w3480:string, after substring=w3479:string)  [unwired: 1 in, 2 out]
                  "bs" <- w3480
                  "as" <- w3479
                  n2349 = Concatenate Strings(w3480, w3479) -> (w3476:string)
                  n2350 = property on="Humidity after test 2" class="DigNum (strict)"("Caption.Text"=w3476) -> ()  [unwired: 2 in, 2 out]
                  n2351 = Concatenate Strings(w3476, "=" ("string")) -> (w3478:string)
                  n2352 = property on="Humidity after test" class="DigNum (strict)"("Caption.Text"=w3476) -> ()  [unwired: 2 in, 2 out]
                  n2353 = local write "S 39"(w3478) -> ()
                }
                frame 39 {
                  n2354 = Match Pattern(string=w3488, regular expression=",") -> (before substring=w3487:string, after substring=w3486:string)  [unwired: 1 in, 2 out]
                  "bs" <- w3487
                  "as" <- w3486
                  n2355 = Concatenate Strings(w3487, w3486) -> (w3483:string)
                  n2356 = property on="Temperature before test 2" class="DigNum (strict)"("Caption.Text"=w3483) -> ()  [unwired: 2 in, 2 out]
                  n2357 = property on="Temperature before test" class="DigNum (strict)"("Caption.Text"=w3483) -> ()  [unwired: 2 in, 2 out]
                  n2358 = Concatenate Strings(w3483, "=" ("string")) -> (→"String 34":string)
                }
                frame 40 {
                  n2359 = Match Pattern(string=w3495, regular expression=",") -> (before substring=w3494:string, after substring=w3493:string)  [unwired: 1 in, 2 out]
                  "bs" <- w3494
                  "as" <- w3493
                  n2360 = Concatenate Strings(w3494, w3493) -> (w3490:string)
                  n2361 = property on="Temperature after test 2" class="DigNum (strict)"("Caption.Text"=w3490) -> ()  [unwired: 2 in, 2 out]
                  n2362 = Concatenate Strings(w3490, "=" ("string")) -> (→"String 35":string)
                  n2363 = property on="Temperature after test" class="DigNum (strict)"("Caption.Text"=w3490) -> ()  [unwired: 2 in, 2 out]
                }
                frame 41 {
                  n2364 = property on="AVP" class="DigNum (strict)"("Caption.Text"=w3499) -> ()  [unwired: 2 in, 2 out]
                  n2365 = property on="AVP 2" class="DigNum (strict)"("Caption.Text"=w3499) -> ()  [unwired: 2 in, 2 out]
                  n2366 = Concatenate Strings(w3499, "=" ("string")) -> (→"String 36":string)
                }
                frame 42 {
                  n2367 = property on="MWSD" class="DigNum (strict)"("Caption.Text"=w3502) -> ()  [unwired: 2 in, 2 out]
                  n2368 = property on="MWSD 2" class="DigNum (strict)"("Caption.Text"=w3502) -> ()  [unwired: 2 in, 2 out]
                  n2369 = Concatenate Strings(w3502, "=" ("string")) -> (→"String 37":string)
                }
                frame 43 {
                  n2370 = property on="HCF 2" class="DigNum (strict)"("Caption.Text"=w3505) -> ()  [unwired: 2 in, 2 out]
                  n2371 = property on="HCF" class="DigNum (strict)"("Caption.Text"=w3505) -> ()  [unwired: 2 in, 2 out]
                  n2372 = Concatenate Strings(w3505, "=" ("string")) -> (→"String 38":string)
                }
                frame 44 {
                  n2373 = Concatenate Strings(w3507, "=" ("string")) -> (→"String 39":string)
                  n2374 = property on="WS1.4 2" class="DigNum (strict)"("Caption.Text"=w3507) -> ()  [unwired: 2 in, 2 out]
                  n2375 = property on="WS1.4" class="DigNum (strict)"("Caption.Text"=w3507) -> ()  [unwired: 2 in, 2 out]
                }
                frame 45 {
                  n2376 = property on="Save Results" class="Bool (strict)"("Boolean Text.Text"=w3509) -> ()  [unwired: 2 in, 2 out]
                }
                frame 46 {
                  n2377 = local write "S 47"(w3510) -> ()
                }
                frame 47 {
                  n2378 = local write "S 48"(w3511) -> ()
                }
                frame 48 {
                  n2379 = local write "S 49"(w3512) -> ()
                }
                frame 49 {
                  n2380 = local write "S 50"(w3513) -> ()
                }
                frame 50 {
                  n2381 = local write "S 51"(w3514) -> ()
                }
                frame 51 {
                  n2382 = local write "S 52"(w3515) -> ()
                }
                frame 52 {
                  n2383 = local write "S 53"(w3516) -> ()
                }
                frame 53 {
                  n2384 = local write "S 54"(w3517) -> ()
                }
                frame 54 {
                  n2385 = local write "S 55"(w3518) -> ()
                }
                frame 55 {
                  n2386 = local write "S 56"(w3519) -> ()
                }
                frame 56 {
                  n2387 = local write "S 57"(w3520) -> ()
                }
                frame 57 {
                  n2388 = local write "S 58"(w3521) -> ()
                }
                frame 58 {
                  n2389 = local write "S 59"(w3522) -> ()
                }
                frame 59 {
                  n2390 = local write "S 60"(w3523) -> ()
                }
                frame 60 {
                  n2391 = local write "S 62"(w3524) -> ()
                }
                frame 61 {
                  n2392 = local write "S 63"(w3525) -> ()
                }
                frame 62 {
                  n2393 = local write "S 64"(w3526) -> ()
                }
                frame 63 {
                  n2394 = local write "S 65"(w3527) -> ()
                }
                frame 64 {
                  n2395 = local write "S 66"(w3528) -> ()
                }
                frame 65 {
                  n2396 = local write "S 67"(w3529) -> ()
                }
                frame 66 {
                  n2397 = local write "S 68"(w3530) -> ()
                }
                frame 67 {
                  n2398 = local write "S 69"(w3531) -> ()
                }
                frame 68 {
                  n2399 = local write "S 70"(w3532) -> ()
                }
                frame 69 {
                  n2400 = local write "S 71"(w3533) -> ()
                }
                frame 70 {
                  n2401 = local write "S 72"(w3534) -> ()
                }
                frame 71 {
                  n2402 = local write "S 73"(w3535) -> ()
                }
                frame 72 {
                  n2403 = local write "S 74"(w3536) -> ()
                }
                frame 73 {
                  n2404 = local write "S 75"(w3537) -> ()
                }
                frame 74 {
                  n2405 = local write "S 76"(w3538) -> ()
                }
                frame 75 {
                  n2406 = local write "S 77"(w3539) -> ()
                }
                frame 76 {
                  n2407 = local write "S 78"(w3540) -> ()
                }
                frame 77 {
                  n2408 = local write "S 79"(w3541) -> ()
                }
                frame 79 {
                  n2409 = property on="Sample Temperature" class="XYGraph (strict)"("Y Scale.Name Label.Text"=w3542) -> ()  [unwired: 2 in, 2 out]
                }
                frame 80 {
                  n2410 = local write "S 81"(w3543) -> ()
                  n2411 = property on="Humidity" class="XYGraph (strict)"("Y Scale.Name Label.Text"=w3543) -> ()  [unwired: 2 in, 2 out]
                }
                frame 78 {
                  n2412 = property on="Air Temperature" class="XYGraph (strict)"("X Scale.Name Label.Text"=w3544) -> ()  [unwired: 2 in, 2 out]
                  n2413 = property on="Humidity" class="XYGraph (strict)"("X Scale.Name Label.Text"=w3544) -> ()  [unwired: 2 in, 2 out]
                  n2414 = property on="Sample Temperature" class="XYGraph (strict)"("X Scale.Name Label.Text"=w3544) -> ()  [unwired: 2 in, 2 out]
                  n2415 = property on="Coefficient Of Friction" class="XYGraph (strict)"("X Scale.Name Label.Text"=w3544) -> ()  [unwired: 2 in, 2 out]
                }
                frame 81 {
                  n2416 = property on="Air Temperature" class="XYGraph (strict)"("Y Scale.Name Label.Text"=w3545) -> ()  [unwired: 2 in, 2 out]
                }
                frame 82 {
                  n2417 = local write "S 84"(w3546) -> ()
                }
                frame 83 {
